vi "readCustomDeviceVersionFromXML.vi"   [LabVIEW 2015, in "nipkg-utilities.lvlib"]
uses:
  nipkg-utilities.lvlib
  <vilib>/xml/Load XML File.vi
  <vilib>/xml/Close Reference(Node).vi
  <vilib>/xml/NI_XML.lvlib
  <vilib>/Wiresmith Technology/LabVIEW CLI/CLI Class/CLI.lvclass
types:
  T1 = enum16{"open", "replace", "create", "open or create", "replace or create", "replace or create with confirmation"}
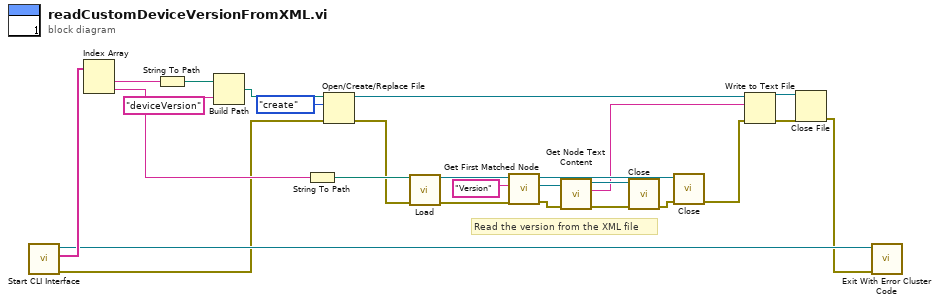
[diagram p0: block diagram]
diagram:
  # "Read the version from the XML file"
  n1 = call <vilib>:"Start CLI Interface.vi"() -> ("error out"=w13:errorcluster, "Custom Parameters"=w17:string[], "CLI out"=w15:refnum<class "CLI.lvclass">)  [unwired: 9 in]
  n2 = Index Array(array=w17) -> (element #1=w12:string, element #2=w14:string)  [unwired: 2 in]
  n3 = String To Path(string=w12) -> (path=w11:path)
  n4 = Build Path(base path=w11, name or relative path="deviceVersion") -> (appended path=w9:path)
  n5 = String To Path(string=w14) -> (path=w18:path)
  n6 = Open/Create/Replace File(file path (use dialog)=w9, error in=w13, operation (0:open)=T1."create") -> (refnum out=w4:refnum<file>, error out=w7:errorcluster)  [unwired: 3 in, 1 out]
  n7 = call-poly <vilib>:"Load.vi"("path to XML document"=w18, "error in (no error)"=w7) -> ("DOM document out"=w24:refnum<k20>, "error out"=w23:errorcluster)  [unwired: 11 in, 1 out]
  n8 = call <vilib>:"Get First Matched Node.vi"("error in (no error)"=w23, "XPath expression"="Version", "node in"=w24) -> ("error out"=w26:errorcluster, "node result"=w25:refnum<k20>, "node out"=w20:refnum<k20>)  [unwired: 6 in]
  n9 = call <vilib>:"Get Node Text Content.vi"("error in (no error)"=w26, "node in"=w25) -> ("error out"=w21:errorcluster, "node text"=w5:string, "node out"=w22:refnum<k20>)  [unwired: 7 in]
  n10 = call-poly <vilib>:"Close.vi"("error in (no error)"=w21, "node"=w22) -> ("error out"=w19:errorcluster)  [unwired: 7 in]
  n11 = call-poly <vilib>:"Close.vi"("error in (no error)"=w19, "node"=w20) -> ("error out"=w6:errorcluster)  [unwired: 7 in]
  n12 = Write to Text File(file (use dialog)=w4, text=w5, error in=w6) -> (refnum out=w3:refnum<file>, error out=w2:errorcluster)  [unwired: 1 in, 1 out]
  n13 = Close File(refnum=w3, error in=w2) -> (error out=w1:errorcluster)  [unwired: 1 out]
  n14 = call <vilib>:"Exit With Error Cluster Code.vi"("error in (no error)"=w1, "CLI in"=w15) -> ()  [unwired: 9 in, 1 out]
